vi "2D array.vi"() -> ()   [LabVIEW 2017]
panel:
  out "Array":dbl[][](array[numeric])
  in  "path 2":path
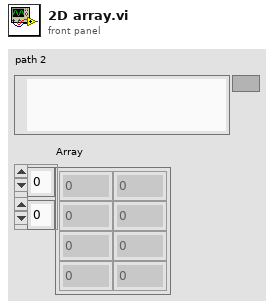
[diagram p1: front panel]
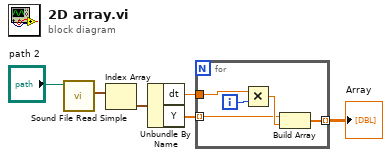
[diagram p0: block diagram]
diagram:
  n1 = call <vilib>:"Sound File Read Simple.vi"("path"="path 2") -> ("data"=w5:waveform(dbl)[])  [unwired: 7 in, 3 out]
  n2 = Index Array(array=w5) -> (element=w4:waveform(dbl))  [unwired: 1 in]
  n3 = Unbundle By Name(w4) -> ("dt"=w3:dbl, "Y"=w2:dbl[])
  n4 = for {
    tunnel: w3 -> [w11]
    tunnel: w2 -> [w8] mode=indexing
    tunnel: [w7] -> w1 mode=indexing
    i -> [w10]
    n5 = Multiply(x=w11, y=w10) -> (x*y=w9:dbl)
    n6 = Build Array(w8, w9) -> (w7:dbl[])
  }
  "Array" <- w1
